vi "Clear GPIB Timeout.vi"(6 "Errors to skip":i32[](array[numeric])=[6, -1073807339, -1073807253, -1073807194], 8 "error in (no error)":errorcluster) -> (0 "error out":errorcluster)   [LabVIEW 2015]
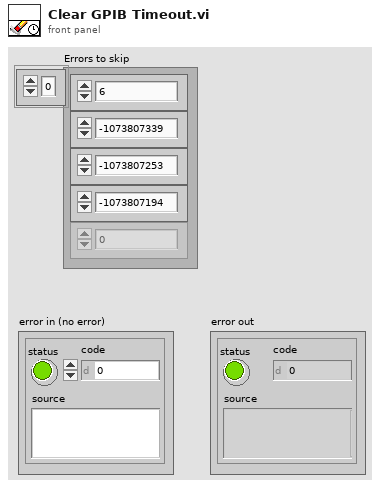
[diagram p1: front panel]
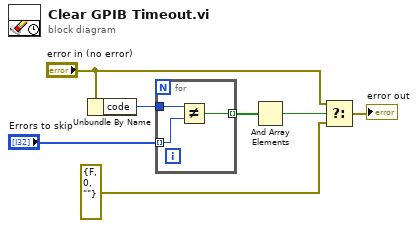
[diagram p0: block diagram]
diagram:
  n1 = Unbundle By Name("error in (no error)") -> ("code"=w7:i32)
  n2 = for {
    tunnel: w7 -> [w10]
    tunnel: [w9] -> w3 mode=indexing
    tunnel: "Errors to skip" -> [w8] mode=indexing
    n3 = Not Equal?(x=w10, y=w8) -> (x != y?=w9:bool)
  }
  n4 = And Array Elements(Boolean array=w3) -> (logical AND=w2:bool)
  n5 = Select(t="error in (no error)", s=w2, f=errorcluster {"status"=FALSE, "code"=0, "source"=""} ("error out")) -> (s? t:f=→"error out":errorcluster)
